vi "General setup-format and values.vi"() -> (14 "DBL":T1, 15 "DBL values":dbl[](array[numeric]), 16 "String":T2, 17 "String values":string[](array[string]), 18 "Boolean":T3, 19 "Boolean values":bool[](array[boolean]))   [LabVIEW 2020]
uses:
  Typedefs/Ini file interface (Boolean).ctl
  Typedefs/Ini file interface (String).ctl
  Typedefs/Ini file interface (DBL).ctl
  Typedefs/fgv_actions.ctl
  Global Variables/General Globals.vi
  Calibration/Globals/gl_Calibration globals.vi
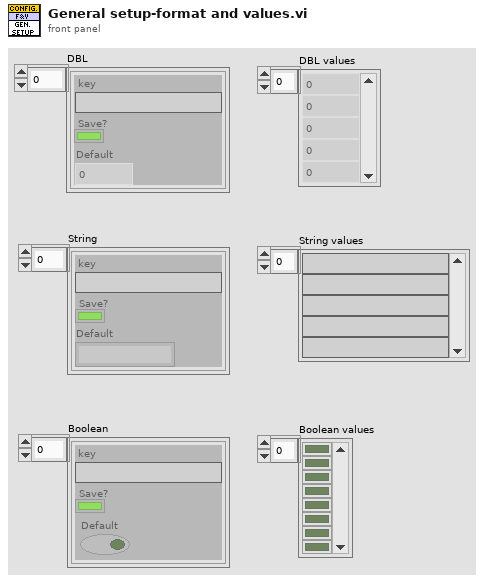
[diagram p1: front panel]
types:
  T1 = typedef "Ini file interface (DBL).ctl" = cluster{"key":string, "Save?":bool, "Default":dbl}[]
  T2 = typedef "Ini file interface (String).ctl" = cluster{"key":string, "Save?":bool, "Default":string}[]
  T3 = typedef "Ini file interface (Boolean).ctl" = cluster{"key":string, "Save?":bool, "Default":bool}[]
  T4 = typedef "fgv_actions.ctl" = enum16{"Get", "Set"}
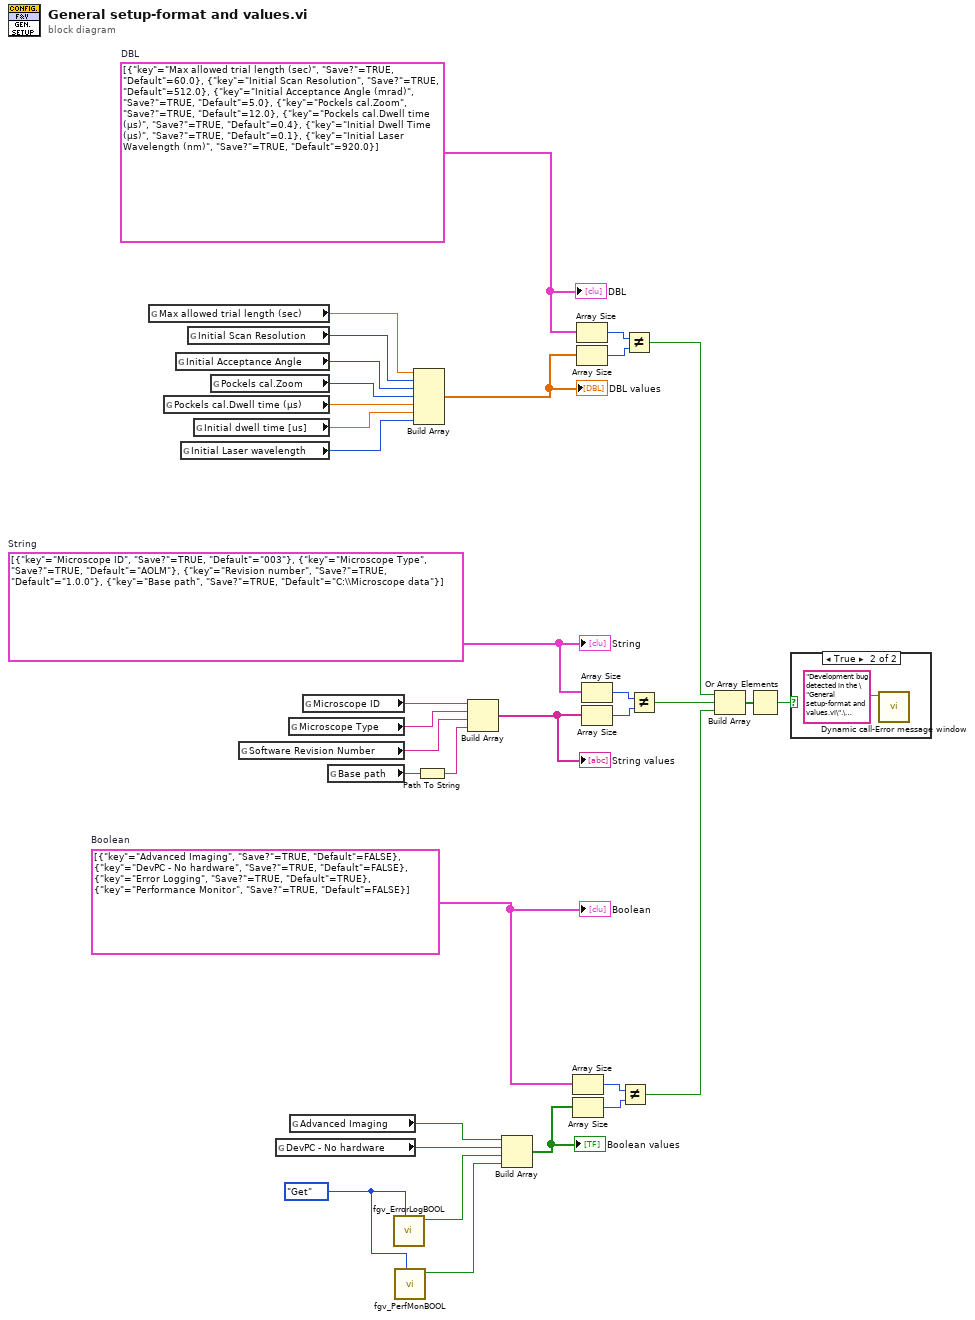
[diagram p0: block diagram]
diagram:
  w4 = fgv_actions."Get" ("FGV Actions")
  w14 = T1 [{"key"="Max allowed trial length (sec)", "Save?"=TRUE, "Default"=60.0}, {"key"="Initial Scan Resolution", "Save?"=TRUE, "Default"=512.0}, {"key"="Initial Acceptance Angle (mrad)", "Save?"=TRUE, "Default"=5.0}, {"key"="Pockels cal.Zoom", "Save?"=TRUE, "Default"=12.0}, {"key"="Pockels cal.Dwell time (µs)", "Save?"=TRUE, "Default"=0.4}, {"key"="Initial Dwell Time (µs)", "Save?"=TRUE, "Default"=0.1}, {"key"="Initial Laser Wavelength (nm)", "Save?"=TRUE, "Default"=920.0}]  # DBL
  w19 = T3 [{"key"="Advanced Imaging", "Save?"=TRUE, "Default"=FALSE}, {"key"="DevPC - No hardware", "Save?"=TRUE, "Default"=FALSE}, {"key"="Error Logging", "Save?"=TRUE, "Default"=TRUE}, {"key"="Performance Monitor", "Save?"=TRUE, "Default"=FALSE}]  # Boolean
  w23 = T2 [{"key"="Microscope ID", "Save?"=TRUE, "Default"="003"}, {"key"="Microscope Type", "Save?"=TRUE, "Default"="AOLM"}, {"key"="Revision number", "Save?"=TRUE, "Default"="1.0.0"}, {"key"="Base path", "Save?"=TRUE, "Default"="C:\\Microscope data"}]  # String
  n1 = global read "General Globals.vi" "Max allowed trial length (sec)"() -> (w31:dbl)
  n2 = global read "gl_Calibration globals.vi" "Pockels cal.Dwell time (µs)"() -> (w12:dbl)
  n3 = global read "General Globals.vi" "Initial Acceptance Angle"() -> (w10:i32)
  n4 = global read "General Globals.vi" "Initial Laser wavelength"() -> (w1:i32)
  n5 = global read "General Globals.vi" "Initial Scan Resolution"() -> (w11:i32)
  n6 = global read "General Globals.vi" "Initial dwell time [us]"() -> (w2:dbl)
  n7 = global read "gl_Calibration globals.vi" "Pockels cal.Zoom"() -> (w13:u8)
  n8 = global read "General Globals.vi" "Software Revision Number"() -> (w7:string)
  n9 = global read "General Globals.vi" "DevPC - No hardware"() -> (w34:bool)
  n10 = global read "General Globals.vi" "Microscope Type"() -> (w8:string)
  n11 = global read "General Globals.vi" "Advanced Imaging"() -> (w6:bool)
  n12 = global read "General Globals.vi" "Microscope ID"() -> (w9:string)
  n13 = global read "General Globals.vi" "Base path"() -> (w32:path)
  n14 = call "fgv_ErrorLogBOOL.vi"("FGV Actions"=w4) -> ("Error Logging ON [OUT]"=w5:bool)  [unwired: 9 in, 1 out]
  n15 = call "fgv_PerfMonBOOL.vi"("FGV Actions"=w4) -> ("Perf Mon [OUT]"=w3:bool)  [unwired: 9 in, 1 out]
  n16 = Build Array(w31, w11, w10, w13, w12, w2, w1) -> (w26:dbl[])
  "DBL values" <- w26
  n17 = Path To String(path=w32) -> (string=w33:string)
  n18 = Build Array(w9, w8, w7, w33) -> (w22:string[])
  "String values" <- w22
  n19 = Build Array(w6, w34, w5, w3) -> (w18:bool[])
  "Boolean values" <- w18
  n20 = Array Size(array=w19) -> (size(s)=w21:i32)
  n21 = Array Size(array=w18) -> (size(s)=w20:i32)
  n22 = Array Size(array=w14) -> (size(s)=w30:i32)
  n23 = Array Size(array=w26) -> (size(s)=w29:i32)
  n24 = Array Size(array=w23) -> (size(s)=w24:i32)
  n25 = Array Size(array=w22) -> (size(s)=w25:i32)
  n26 = Not Equal?(x=w21, y=w20) -> (x != y?=w15:bool)
  n27 = Not Equal?(x=w30, y=w29) -> (x != y?=w17:bool)
  n28 = Not Equal?(x=w24, y=w25) -> (x != y?=w16:bool)
  n29 = Build Array(w17, w16, w15) -> (w28:bool[])
  n30 = Or Array Elements(Boolean array=w28) -> (logical OR=w27:bool)
  n31 = case shown="True" w27 {
    frame False {
    }
    frame True {
      n32 = call "Dynamic call-Error message window.vi"("Error Message"="Development bug detected in the \"General setup-format and values.vi\".\nPlease correct the set up in this VI.") -> ()  [unwired: 10 in, 1 out]
    }
  }
  "Boolean" <- w19
  "String" <- w23
  "DBL" <- w14
